vi "Locate Target.vi"() -> ()   [LabVIEW 2013]
uses:
  <vilib>/vision/NI_Vision_Development_Module.lvlib
panel:
  out "Bird":u32[][](graph)
  out "Image":u8[][](graph)
  out "y":sgl
  out "x":sgl
  out "Template":u8[][](graph)
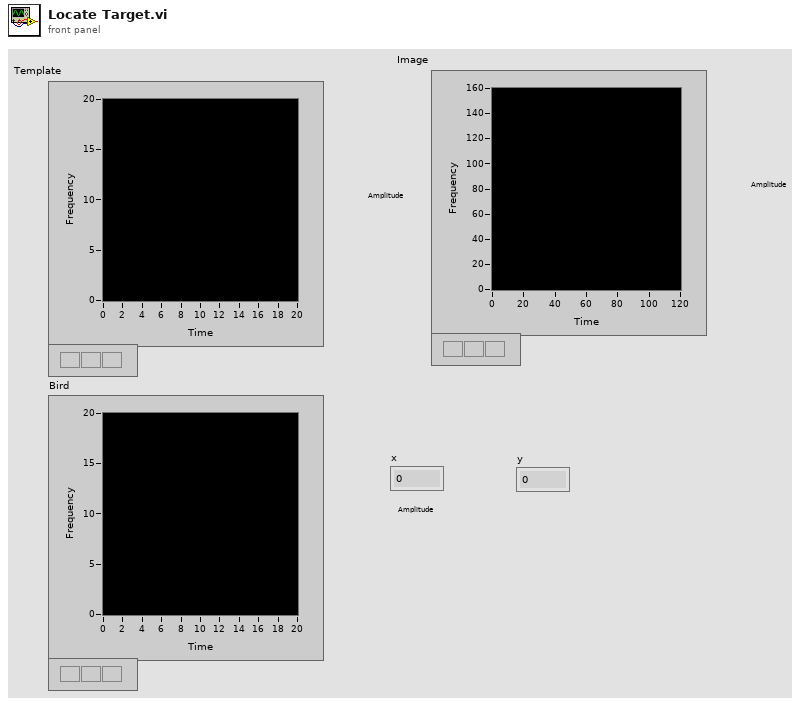
[diagram p1: front panel]
types:
  T1 = typedef "IMAQ Image.ctl" = refnum<image>
  T2 = cluster{"Position":cluster{"x":sgl, "y":sgl}, "Angle":sgl, "Scale":sgl, "Score":sgl, "Bounding Box":cluster{"x":sgl, "y":sgl}[]}[]
  T3 = cluster{"Position":cluster{"x":sgl, "y":sgl}, "Angle":sgl, "Scale":sgl, "Score":sgl, "Bounding Box":cluster{"x":sgl, "y":sgl}[]}
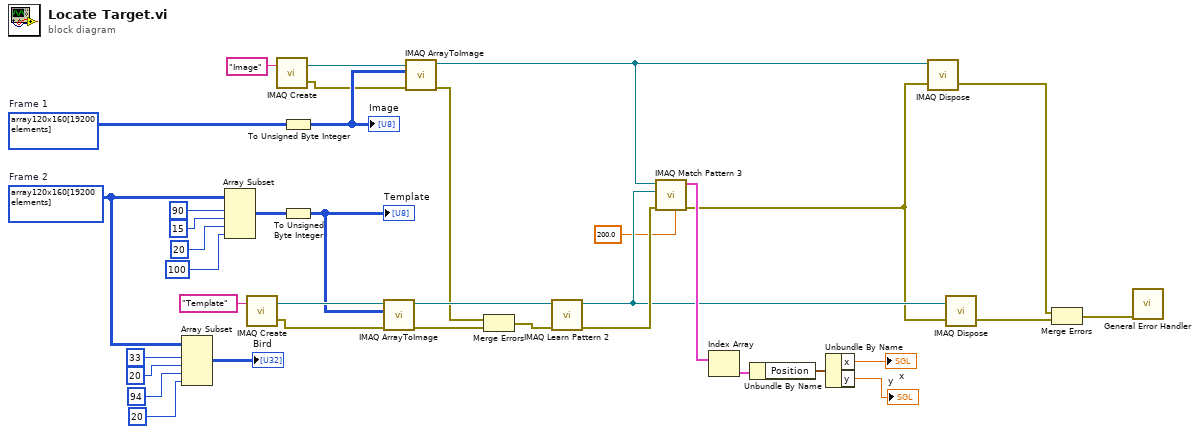
[diagram p0: block diagram]
diagram:
  w3 = u32[][] array120x160[19200 elements]  # Frame 2
  w23 = u32[][] array120x160[19200 elements]  # Frame 1
  n1 = Array Subset(array=w3, index (row)=33 ("index"), length (row)=20 ("length"), index (col)=94 ("index"), length (col)=20 ("length")) -> (→"Bird":u32[][])
  n2 = Array Subset(array=w3, index (row)=90 ("index"), length (row)=15 ("length"), index (col)=20 ("index"), length (col)=100 ("length")) -> (w1:u32[][])
  n3 = call "IMAQ Create"("Image Name"="Template") -> ("New Image"=w31:T1, "error out"=w20:errorcluster)  [unwired: 4 in]
  n4 = call "IMAQ Create"("Image Name"="Image") -> ("New Image"=w37:T1, "error out"=w21:errorcluster)  [unwired: 4 in]
  n5 = To Unsigned Byte Integer(number=w23) -> (unsigned 8bit integer=w24:u8[][])
  "Image" <- w24
  n6 = To Unsigned Byte Integer(number=w1) -> (unsigned 8bit integer=w9:u8[][])
  "Template" <- w9
  n7 = call "IMAQ ArrayToImage"("error in (no error)"=w20, "Image Pixels (U8)"=w9, "Image"=w31) -> ("error out"=w19:errorcluster, "Image Out"=w30:T1)  [unwired: 7 in]
  n8 = call "IMAQ ArrayToImage"("error in (no error)"=w21, "Image Pixels (U8)"=w24, "Image"=w37) -> ("error out"=w16:errorcluster, "Image Out"=w22:T1)  [unwired: 7 in]
  n9 = Merge Errors(w16, w19) -> (w17:errorcluster)
  n10 = call "IMAQ Learn Pattern 2"("error in (no error)"=w17, "Image"=w30) -> ("error out"=w18:errorcluster, "Template Image Out"=w15:T1)  [unwired: 8 in]
  n11 = call "IMAQ Match Pattern 3"("Minimum Match Score"=sgl 200.0, "error in (no error)"=w18, "Template Image"=w15, "Image"=w22) -> ("error out"=w14:errorcluster, "Matches"=w27:T2)  [unwired: 5 in, 1 out]
  n12 = Index Array(array=w27) -> (element=w29:T3)  [unwired: 1 in]
  n13 = Unbundle By Name(w29) -> ("Position"=w28:cluster{"x":sgl, "y":sgl})
  n14 = Unbundle By Name(w28) -> ("x"=→"x":sgl, "y"=→"y":sgl)
  n15 = call "IMAQ Dispose"("Image"=w22, "error in (no error)"=w14) -> ("error out"=w12:errorcluster)  [unwired: 4 in]
  n16 = call "IMAQ Dispose"("Image"=w15, "error in (no error)"=w14) -> ("error out"=w13:errorcluster)  [unwired: 4 in]
  n17 = Merge Errors(w12, w13) -> (w11:errorcluster)
  n18 = call <vilib>:"General Error Handler.vi"("error in (no error)"=w11) -> ()  [unwired: 10 in, 5 out]
